vi "3220_Cde_Serial.vi"(6 "Chaîne à écrire":string="0 CURR MES\r", 8 "error in":errorcluster, 11 "VISA In":refnum<visa-resource-name>="COM3") -> (0 "error out":errorcluster, 1 "Message d'erreur":string, 2 "Réponse":string="0 OK 994\r", 3 "Nombre d'octets lus":u32=9)   [LabVIEW 2020]
doc: "Commande basique de l'<B>ALR 3220:</B>\nInitialisation, écriture, lecture, traitement mise en garde, fermeture port.\n\n<B>Note:</B>\nLe protocole de communication est joint sur la face avant."
uses:
  <vilib>/Utility/error.llb/DialogType.ctl
panel:
  # "Interprétation de LabVIEW\nValeur hexadécimale d'un caractère 8 bits, qui doit être en majuscule\nRetour arrière ( ASCII BS, correspondant à \\08 )\nSaut de page ( ASCII FF, correspondant à \\0C )\nSaut de ligne ( ASCII LF, correspondant à \\0A ) — La fonction Formater dans un fichier convertit automatiquement ce code en caractère de fin de ligne dépendant de la plate-forme.\nRetour chariot ( ASCII CR, correspondant à \\0D )\nTabulation ( ASCII HT, correspondant à \\09 )\nEspace ( correspondant à \\20 )\nBarre oblique inverse ( ASCII \\, correspondant à \\5C )\nPour cent"
  # "SYNTAXE DE COMMUNICATION DE l'ALR3220\nFormat des commandes :\nAdresse <space>Paramètre<space>Commande[<space>Valeur]<CR>\nExemple 0 VOLT WR 1256\nExemple 1 CURR MES\n\nRéponse :\nAdresse <space>Status<space>Valeur<CR>\nRetour de réponse après exécution\nExemple : 0 ERR 8\nExemple : 1 OK 456 8\n\nListe des Paramètres :\nVOLT => Tension de sortie (0 à 32100 mV)\nCURR => Courant de sortie (0 à 20450 mA)\nOVP  => Tension maximum de sortie (0 à 32100 mV)\nOCP  => Courant maximum de sortie (0 à 32100 mV)\nRCL  => Rappel configuration (1 à 16)\nSTO  => Sauvegarde configuration (0 à 16)\nOUT => ON/OFF (0 = OFF, >=1 ON)\n\nListe des Commandes :\nWR => Ecriture consigne (Valable pour tous les paramètres)\nRD => Lecture consigne (Valide pour tous sauf paramètres RCL & STO)\nMES  => Lecture mesure (Valide uniquement pour paramètres VOLT & CURR)"
  # "This V.I was designed to control the ALR3220, it can be adapted as is to order the ALR3203 \n(Pmax = 96W). To order the ALR3206 D & T, just add the Channel number following the \nparameters. Ex: I want 20V on channel 2: 0 VOLT2 WR 20000"
  # "Ce V.I a été concu pourcontrôler l'ALR3220, il peut être  adapté tel-quel pour commander \nl'ALR3203 (Pmax = 96W). Pour commander les ALR3206 D & T, il suffit de rajouter le \nN° de la voie à la suite des paramètres. Ex : Je veux 20V sur la voie 2 : 0 VOLT2 WR 20000"
  # "© 2008 2020 ELC  ALL RIGHTS RESERVED."
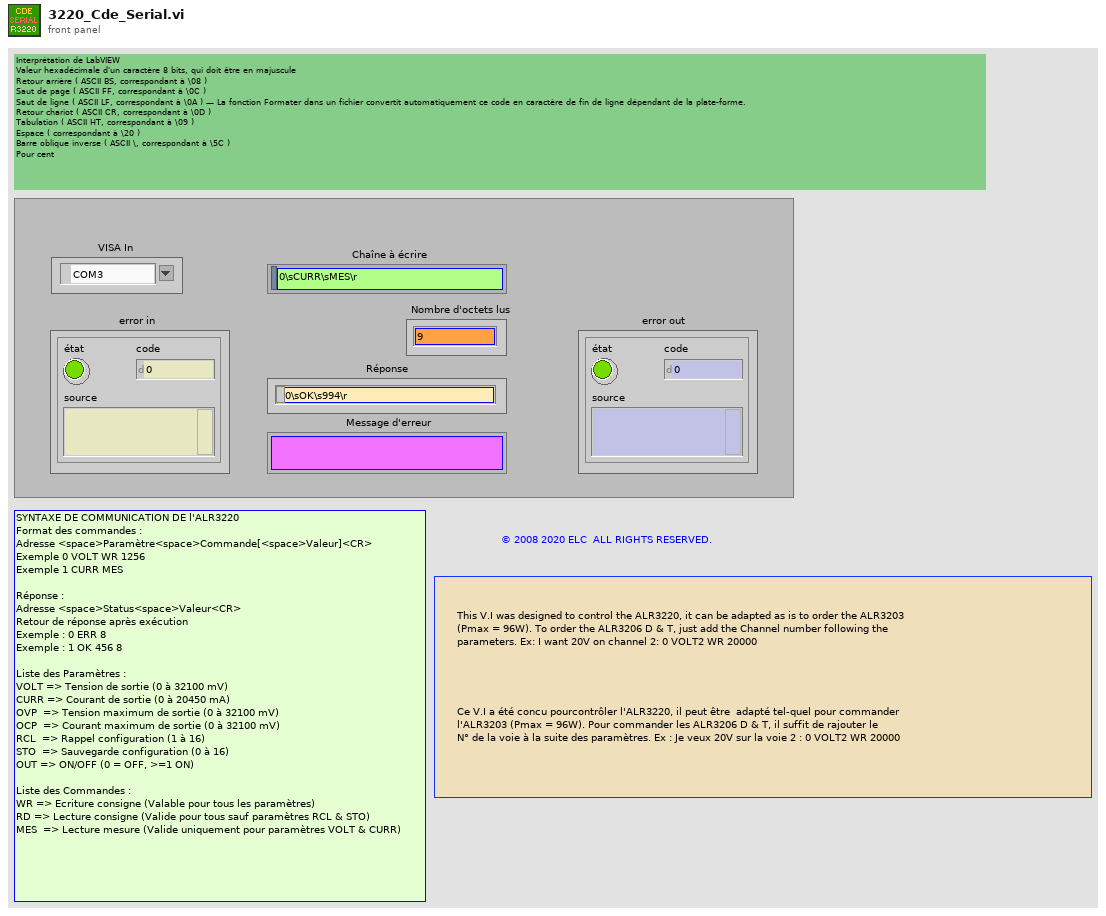
[diagram p1: front panel]
types:
  T1 = typedef "DialogType.ctl" = u16
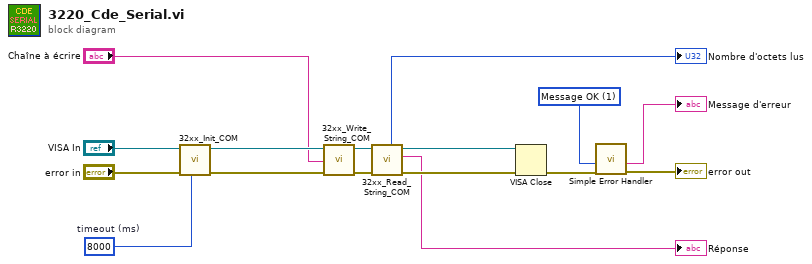
[diagram p0: block diagram]
diagram:
  w6 = T1 1 items=["pas de dialogue", "Message OK", "Message continuer ou arrêter", "Message OK + mises en garde", "Arrêter/Continuer + mises en garde"] ("type of dialog (OK msg:1)")
  w16 = u32 8000  # timeout (ms)
  n1 = call "32xx_Init_COM.vi"("Time\nOut (ms)"=w16, "Entrée d'erreur"="error in", "Port d'entrée"="VISA In") -> ("Sortie d'erreur"=w13:errorcluster, "Port de sortie"=w14:refnum<visa-resource-name>)  [unwired: 6 in, 1 out]
  n2 = call "32xx_Write_String_COM.vi"("Chaîne à écrire"="Chaîne à écrire", "entrée d'erreur"=w13, "Port d'entrée"=w14) -> ("sortie d'erreur"=w2:errorcluster, "Port de sortie"=w1:refnum<visa-resource-name>)  [unwired: 7 in]
  n3 = call "32xx_Read_String_COM.vi"("entrée d'erreur"=w2, "Port d'entrée"=w1) -> ("Sortie d'erreur"=w10:errorcluster, "Réponse"=→"Réponse":string, "Port de sortie"=w9:refnum<visa-resource-name>, "octets lus"=→"Nombre d'octets lus":u32)  [unwired: 6 in]
  n4 = VISA Close(VISA resource name=w9, error in (no error)=w10) -> (error out=w5:errorcluster)
  n5 = call <vilib>:"Simple Error Handler.vi"("type of dialog (OK msg:1)"=w6, "error in (no error)"=w5) -> ("source out"=→"Message d'erreur":string, "error out"=→"error out":errorcluster)  [unwired: 6 out]
